vi "Read Range from Scene.vi"(6 "Control Ref Queue":T1, 8 "error in (no error)":errorcluster, 10 "Default Range Value":sgl, 11 "Label Object Name":string) -> (0 "error out":errorcluster, 2 "Min":sgl, 3 "Max":sgl)   [LabVIEW 2020, in "3D Plot.lvclass"]
uses:
  3D Plot.lvclass
  3DMathPlot Ctrl Act Queue.ctl
  3DMathPlot Ctrl Act Cluster.ctl
  3DMathPlot State Class.ctl
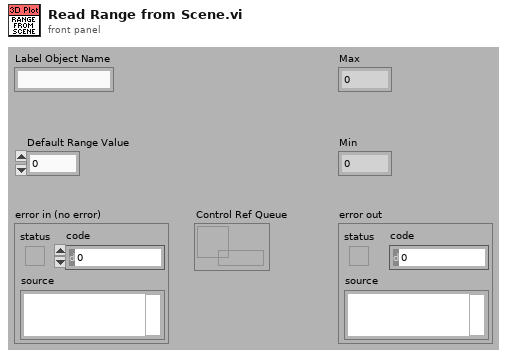
[diagram p1: front panel]
types:
  T1 = typedef "3DMathPlot Ctrl Act Queue.ctl" = refnum<queue>
  T2 = typedef "3DMathPlot Ctrl Act Cluster.ctl" = cluster{"3D Picture Control":refnum<vi>, "Render Window Refnum":refnum<vi>, "XY Graph":refnum<vi>, "Intensity Graph":refnum<vi>, "Color Legend Palette":refnum<vi>, "Projection Palette":refnum<vi>, "XControl  Ref":refnum<vi>, "Facade Ref":refnum<vi>, "Export Image Ref":refnum<vi>, "Clear Data Flag":bool, "Display State Change Class":T3}
  T3 = typedef "3DMathPlot State Class.ctl" = enum16{"Update All Objects (Undo)", "Update Light Object Only", "Update Axis Object Only", "Update Plot Object Only", "Update Cursor Object Only", "Update Axis Plot Cursor Objects", "No Update"}
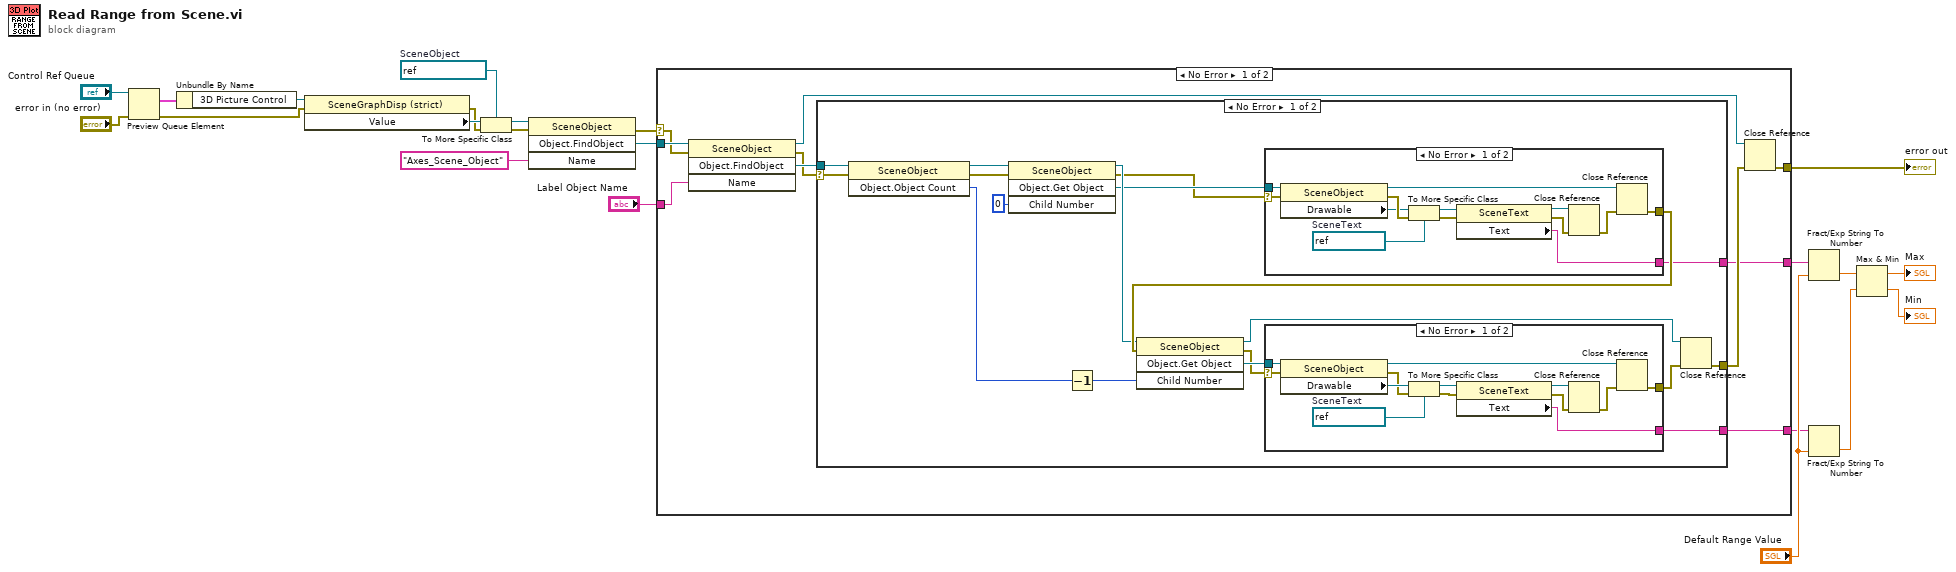
[diagram p0: block diagram]
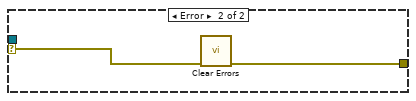
[diagram p2: hidden frame]
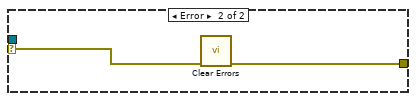
[diagram p3: hidden frame]
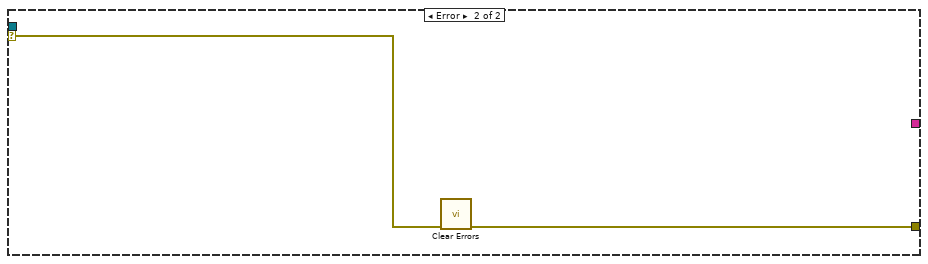
[diagram p4: hidden frame]
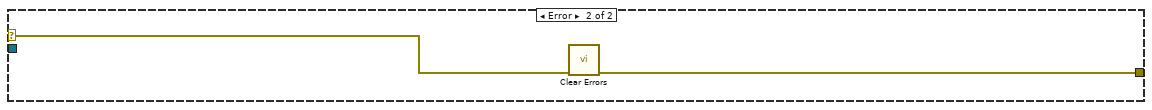
[diagram p5: hidden frame]
diagram:
  w10 = refnum<vi> refnum  # SceneObject
  n1 = Preview Queue Element(queue="Control Ref Queue", error in (no error)="error in (no error)") -> (element=w12:T2, error out=w5:errorcluster)  [unwired: 1 in, 2 out]
  n2 = Unbundle By Name(w12) -> ("3D Picture Control"=w11:refnum<vi>)
  n3 = property class="SceneGraphDisp (strict)"(reference=w11, error in=w5) -> (error out=w4:errorcluster, "Value"=w16:refnum<vi>)  [unwired: 1 out]
  n4 = To More Specific Class(target class=w10, reference=w16, error in=w4) -> (specific class reference=w9:refnum<vi>, error out=w3:errorcluster)
  n5 = invoke class="SceneObject" method="Object.FindObject"(reference=w9, error in=w3, "Name"="Axes_Scene_Object") -> (error out=w1:errorcluster, "FindObject"=w7:refnum<vi>)  [unwired: 1 in, 2 out]
  n6 = case shown="No Error" w1 {
    selector: w1 -> [w24 w84]
    tunnel: [w32 w83] -> w22
    tunnel: [w29 _] -> w17
    tunnel: "Label Object Name" -> [w28 _]
    tunnel: w7 -> [w27 _]
    tunnel: [w25 _] -> w6
    frame No Error {
      n7 = invoke class="SceneObject" method="Object.FindObject"(reference=w27, error in=w24, "Name"=w28) -> (reference out=w30:refnum<vi>, error out=w23:errorcluster, "FindObject"=w26:refnum<vi>)  [unwired: 1 in, 1 out]
      n8 = case shown="No Error" w23 {
        selector: w23 -> [w35 w82]
        tunnel: [w50 w81] -> w31
        tunnel: [w45 _] -> w29
        tunnel: w26 -> [w41 _]
        tunnel: [w38 _] -> w25
        frame No Error {
          n9 = invoke class="SceneObject" method="Object.Object Count"(reference=w41, error in=w35) -> (reference out=w37:refnum<vi>, error out=w36:errorcluster, "Child Count"=w42:i32)  [unwired: 1 in]
          n10 = invoke class="SceneObject" method="Object.Get Object"(reference=w37, error in=w36, "Child Number"=0 ("index")) -> (reference out=w44:refnum<vi>, error out=w34:errorcluster, "Get Child"=w40:refnum<vi>)  [unwired: 1 in, 1 out]
          n11 = Decrement(x=w42) -> (x-1=w43:i32)
          n12 = case shown="No Error" w34 {
            selector: w34 -> [w66 w80]
            tunnel: [w78 w79] -> w47
            tunnel: w40 -> [w70 _]
            tunnel: [w68 _] -> w38
            frame No Error {
              w72 = refnum<vi> refnum  # SceneText
              n13 = property class="SceneObject"(reference=w70, error in=w66) -> (reference out=w76:refnum<vi>, error out=w73:errorcluster, "Drawable"=w71:refnum<vi>)
              n14 = To More Specific Class(target class=w72, reference=w71, error in=w73) -> (specific class reference=w69:refnum<vi>, error out=w67:errorcluster)
              n15 = property class="SceneText"(reference=w69, error in=w67) -> (reference out=w74:refnum<vi>, error out=w75:errorcluster, "Text"=w68:string)
              n16 = Close Reference(reference=w74, error in (no error)=w75) -> (error out=w77:errorcluster)
              n17 = Close Reference(reference=w76, error in (no error)=w77) -> (error out=w78:errorcluster)
            }
            frame Error {
              n18 = call "Clear Errors.vi"("error in (no error)"=w80) -> ("error out"=w79:errorcluster)  [unwired: 5 in, 1 out]
            }
          }
          n19 = invoke class="SceneObject" method="Object.Get Object"(reference=w44, error in=w47, "Child Number"=w43) -> (reference out=w48:refnum<vi>, error out=w33:errorcluster, "Get Child"=w46:refnum<vi>)  [unwired: 1 in, 1 out]
          n20 = case shown="No Error" w33 {
            selector: w33 -> [w51 w65]
            tunnel: [w63 w64] -> w49
            tunnel: w46 -> [w58 _]
            tunnel: [w56 _] -> w45
            frame No Error {
              w53 = refnum<vi> refnum  # SceneText
              n21 = property class="SceneObject"(reference=w58, error in=w51) -> (reference out=w61:refnum<vi>, error out=w52:errorcluster, "Drawable"=w54:refnum<vi>)
              n22 = To More Specific Class(target class=w53, reference=w54, error in=w52) -> (specific class reference=w55:refnum<vi>, error out=w57:errorcluster)
              n23 = property class="SceneText"(reference=w55, error in=w57) -> (reference out=w59:refnum<vi>, error out=w60:errorcluster, "Text"=w56:string)
              n24 = Close Reference(reference=w59, error in (no error)=w60) -> (error out=w62:errorcluster)
              n25 = Close Reference(reference=w61, error in (no error)=w62) -> (error out=w63:errorcluster)
            }
            frame Error {
              n26 = call "Clear Errors.vi"("error in (no error)"=w65) -> ("error out"=w64:errorcluster)  [unwired: 5 in, 1 out]
            }
          }
          n27 = Close Reference(reference=w48, error in (no error)=w49) -> (error out=w50:errorcluster)
        }
        frame Error {
          n28 = call "Clear Errors.vi"("error in (no error)"=w82) -> ("error out"=w81:errorcluster)  [unwired: 5 in, 1 out]
        }
      }
      n29 = Close Reference(reference=w30, error in (no error)=w31) -> (error out=w32:errorcluster)
    }
    frame Error {
      n30 = call "Clear Errors.vi"("error in (no error)"=w84) -> ("error out"=w83:errorcluster)  [unwired: 5 in, 1 out]
    }
  }
  "error out" <- w22
  n31 = Fract/Exp String To Number(string=w6, default (0 dbl)="Default Range Value") -> (number=w19:sgl)  [unwired: 2 in, 1 out]
  n32 = Fract/Exp String To Number(string=w17, default (0 dbl)="Default Range Value") -> (number=w20:sgl)  [unwired: 2 in, 1 out]
  n33 = Max & Min(x=w19, y=w20) -> (max(x,y)=→"Max":sgl, min(x,y)=→"Min":sgl)
